vi "Set IP Address.vi"(7 "Set IP Packet":string, 8 "Input parameter 3":string, 9 "Input parameter 2":string, 10 "Input parameter 1":string, 11 "MAC Address HEX":string) -> (3 "Output frame":string)   [LabVIEW 2017]
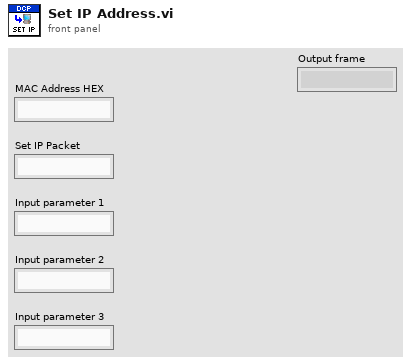
[diagram p1: front panel]
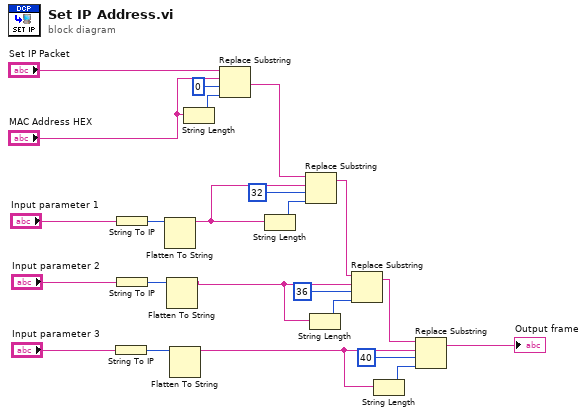
[diagram p0: block diagram]
diagram:
  n1 = String To IP(1:"Input parameter 3") -> (0:w11:u32)
  n2 = String To IP(1:"Input parameter 1") -> (0:w13:u32)
  n3 = String To IP(1:"Input parameter 2") -> (0:w10:u32)
  n4 = Flatten To String(anything=w13) -> (data string=w12:string)  [unwired: 3 in, 2 out]
  n5 = Flatten To String(anything=w10) -> (data string=w3:string)  [unwired: 3 in, 2 out]
  n6 = Flatten To String(anything=w11) -> (data string=w2:string)  [unwired: 3 in, 2 out]
  n7 = String Length(string="MAC Address HEX") -> (length=w22:i32)
  n8 = Replace Substring(2:w22, 3:0 ("offset (0)"), 4:"MAC Address HEX", 5:"Set IP Packet") -> (1:w14:string)  [unwired: 1 out]
  n9 = String Length(string=w12) -> (length=w15:i32)
  n10 = Replace Substring(2:w15, 3:32 ("offset (0)"), 4:w12, 5:w14) -> (1:w7:string)  [unwired: 1 out]
  n11 = String Length(string=w3) -> (length=w8:i32)
  n12 = Replace Substring(2:w8, 3:36 ("offset (0)"), 4:w3, 5:w7) -> (1:w4:string)  [unwired: 1 out]
  n13 = String Length(string=w2) -> (length=w5:i32)
  n14 = Replace Substring(2:w5, 3:40 ("offset (0)"), 4:w2, 5:w4) -> (1:→"Output frame":string)  [unwired: 1 out]
